vi "Check uService Status.vi"(8 "error in (no error)":errorcluster, 10 "uService ID":string, 11 "Ancestor in":refnum<class "Ancestor.lvclass">) -> (0 "error out":errorcluster, 1 "Last Pat":timestamp, 2 "Online?":bool, 3 "Ancestor out":refnum<class "Ancestor.lvclass">)   [LabVIEW 2026, in "TALOS.lvlib" / "Ancestor.lvlib" / "Ancestor.lvclass"]
doc: "This VI check the status of a uService on the local Guardian, returning Online? if correctly running, and when it was last checked."
uses:
  Ancestor.lvclass
  Classes/uService List/uService List.lvclass/uService List.ctl
  Ancestor.lvclass/Ancestor.ctl
  Classes/uService List/Get Last Pat.vi
  Classes/uService List/Get Online Status.vi
  Support VIs/Generate Error.vi
  FGV/Error Memory/Get Error Description.vi
  Support VIs/Get PC name.vi
  Read ID.vi
  Support VIs/Get Class Name.vi
  <vilib>/Utility/error.llb/Clear Errors.vi
  FGV/Error Memory/Error Memory Core.vi
  <vilib>/AdvancedString/Delimited String to 1D String Array.vi
  <vilib>/AdvancedString/Delimited String to 1D String Array (string).vi
  Support VIs/Circus Root Path.vi
  FGV/Error Memory/Error Crt Lvl checker.vi
  FGV/Error Memory/Error Memory Core.vi/40c8088d-b597-4017-91af-faa98e00292e.vi
  FGV/Error Memory/Error Memory Core.vi/d4a3ab98-063c-4e44-b43d-fbdcfe6c2be2.vi
  Support VIs/Global Memory.vi
  <vilib>/Utility/LVClass/Get LV Class Name.vi
  Support VIs/Is in Packed Library.vi
  Support VIs/TALOS Root path.vi
  Support VIs/Read CSV worksheet.vi
  Support VIs/Global Constants.vi
  <vilib>/Utility/error.llb/General Error Handler.vi
  Support VIs/Error Log.vi
  <vilib>/Comparison/Equal/Equal Functor/Equal Functor.lvclass
  Classes/uService List/uService List.lvclass
  TALOS.lvlib
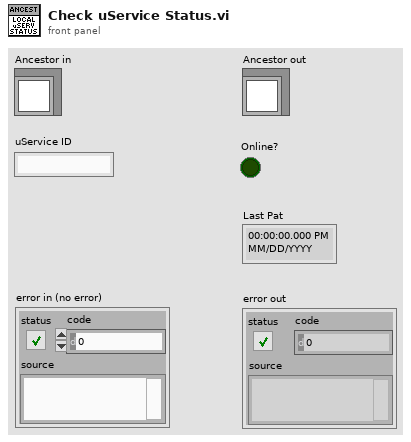
[diagram p1: front panel]
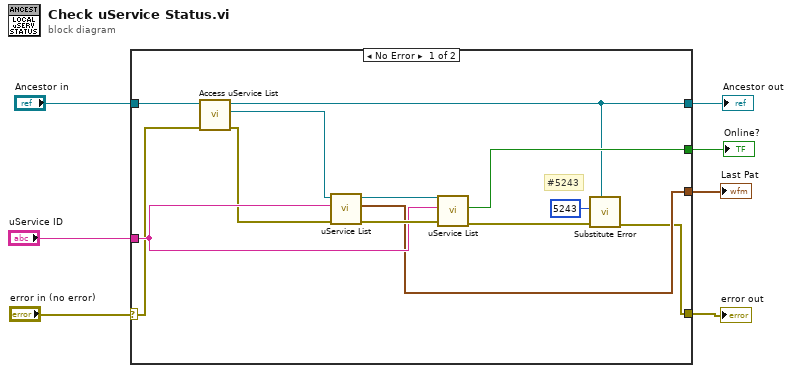
[diagram p0: block diagram]
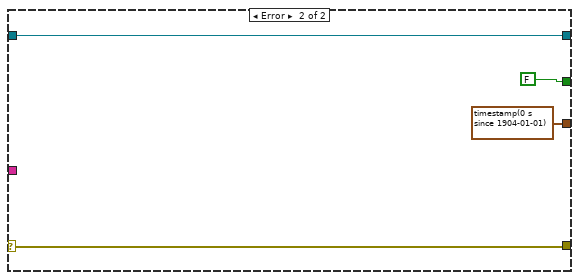
[diagram p2: hidden frame]
diagram:
  n1 = case shown="No Error" "error in (no error)" {
    selector: "error in (no error)" -> [w14 w24]
    tunnel: [w9 w24] -> w7
    tunnel: [w16 FALSE ("Online")] -> w5
    tunnel: [w18 timestamp(0 s since 1904-01-01) ("Last Pat")] -> w4
    tunnel: "uService ID" -> [w19 _]
    tunnel: "Ancestor in" -> [w15 w21]
    tunnel: [w11 w21] -> w1
    frame No Error {
      # "#5243"
      n2 = call-dynamic "Access uService List.vi"("error in (no error)"=w14, "Ancestor in"=w15) -> ("error out"=w13:errorcluster, "uService List out"=w12:refnum<class "uService List.lvclass">, "Ancestor out"=w11:refnum<class "Ancestor.lvclass">)  [unwired: 7 in]
      n3 = call-poly "uService List.vi"("error in (no error)"=w13, "ID"=w19, "uService List in"=w12) -> ("error out"=w20:errorcluster, "Last Pat"=w18:timestamp, "uService List out"=w17:refnum<class "uService List.lvclass">)  [unwired: 6 in]
      n4 = call-poly "uService List.vi"("error in (no error)"=w20, "ID"=w19, "uService List in"=w17) -> ("error out"=w10:errorcluster, "Online"=w16:bool)  [unwired: 6 in, 1 out]
      n5 = call "Substitute Error.vi"("LabVIEW Object"=w11, "error in (no error)"=w10, "Error Code"=5243) -> ("error out"=w9:errorcluster)  [unwired: 8 in]
    }
    frame Error {
    }
  }
  "Online?" <- w5
  "Last Pat" <- w4
  "error out" <- w7
  "Ancestor out" <- w1
